vi "Init Hardware.vi"(8 "error in (no error)":errorcluster, 11 "Ni-Scope Digitizer in":refnum<class "Ni-Scope Digitizer.lvclass">) -> (0 "error out":errorcluster, 3 "Ni-Scope Digitizer out":refnum<class "Ni-Scope Digitizer.lvclass">)   [LabVIEW 2016, in "Ni-Scope Digitizer.lvclass"]
uses:
  Ni-Scope Digitizer.lvclass
  C:/github/NHMFL_Core/Libraries/Instruments/Pulse Driver/Pulse Driver.lvclass
  <instrlib>/niScope/Controls/niScope trigger source digital.ctl
  Ni-Scope Digitizer.lvclass/Ni-Scope Digitizer.ctl
  Instruments/Pulse Driver/Pulse Driver.lvclass/Pulse Driver.ctl
  Read Device name.vi
  Instruments/Pulse Driver/Read Pretrigger samples.vi
  Instruments/Pulse Driver/Read Samples per channel.vi
  Instruments/Pulse Driver/Write Samples per channel.vi
  Instruments/Pulse Driver/Write dt.vi
  Instruments/Pulse Driver/Write t0.vi
  <instrlib>/niScope/Configure/Trigger/niScope Configure Trigger Digital.vi
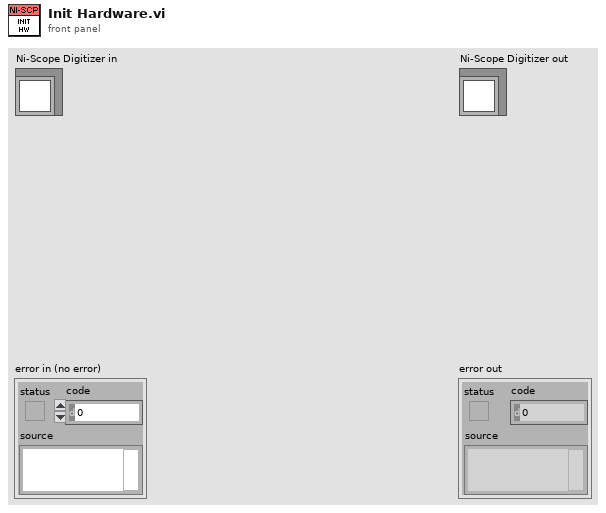
[diagram p1: front panel]
types:
  T1 = typedef "niScope trigger source digital.ctl" = string
  T2 = typedef "Pusle Driver Configuration.ctl" = cluster{"Pre-trigger duration":dbl, "Post-trigger duration":dbl, "Rate":dbl, "Ranges":dbl[], "Re-name channels":string[], "Active channels":string, "External clock":bool}
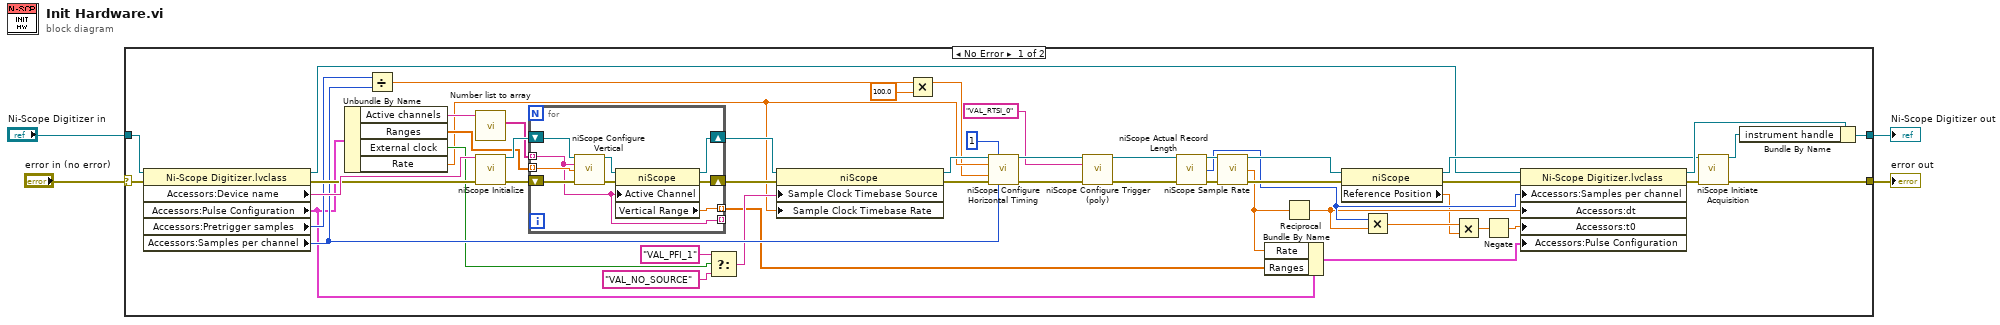
[diagram p0: block diagram]
diagram:
  n1 = case shown="No Error" "error in (no error)" {
    selector: "error in (no error)" -> [w44 w66]
    tunnel: [w8 w66] -> w3
    tunnel: [w14 w65] -> w1
    tunnel: "Ni-Scope Digitizer in" -> [w12 w65]
    frame No Error {
      n2 = property class="Ni-Scope Digitizer.lvclass"(reference=w12, error in=w44) -> (reference out=w11:refnum<class "Ni-Scope Digitizer.lvclass">, error out=w45:errorcluster, "Accessors:Device name"=w46:string, "Accessors:Pulse Configuration"=w26:T2, "Accessors:Pretrigger samples"=w42:u32, "Accessors:Samples per channel"=w43:i32)
      n3 = Unbundle By Name(w26) -> ("Active channels"=w49:string, "Ranges"=w47:dbl[], "External clock"=w37:bool, "Rate"=w33:dbl)
      n4 = Divide(x=w42, y=w43) -> (x/y=w52:dbl)
      n5 = call "Number list to array.vi"("Number list"=w49) -> ("Full names"=w48:string[])  [unwired: 9 in, 1 out]
      n6 = call <instrlib>:"niScope Initialize.vi"("resource name"=w46, "error in"=w45) -> ("instrument handle"=w54:refnum<k15>, "error out"=w55:errorcluster)  [unwired: 2 in, 10 out]
      n7 = for {
        tunnel: w47 -> [w62] mode=indexing
        shift-right: [w58] -> w40
        shift-left: w55 -> [w64]
        shift-right: [w60] -> w41
        shift-left: w54 -> [w63]
        tunnel: w48 -> [w57] mode=indexing
        tunnel: [w57] -> _ mode=indexing
        tunnel: [w56] -> w10 mode=indexing
        n8 = call <instrlib>:"niScope Configure Vertical.vi"("instrument handle"=w63, "channels"=w57, "vertical range"=w62, "error in"=w64) -> ("instrument handle out"=w61:refnum<k15>, "error out"=w59:errorcluster)  [unwired: 10 in]
        n9 = property class="niScope"(reference=w61, error in=w59, "Active Channel"=w57) -> (reference out=w60:refnum<k15>, error out=w58:errorcluster, "Vertical Range"=w56:dbl)
      }
      n10 = Select(t="VAL_PFI_1", s=w37, f="VAL_NO_SOURCE") -> (s? t:f=w34:string)
      n11 = property class="niScope"(reference=w41, error in=w40, "Sample Clock Timebase Source"=w34, "Sample Clock Timebase Rate"=w33) -> (reference out=w39:refnum<k15>, error out=w38:errorcluster)
      n12 = Multiply(x=w52, y=100.0) -> (x*y=w6:dbl)
      n13 = call <instrlib>:"niScope Configure Horizontal Timing.vi"("instrument handle"=w39, "number of records"=1, "min sample rate"=w33, "reference position"=w6, "error in"=w38, "min record length"=w43) -> ("instrument handle out"=w51:refnum<k15>, "error out"=w50:errorcluster)  [unwired: 1 in, 7 out]
      n14 = call-poly <instrlib>:"niScope Configure Trigger (poly).vi"("instrument handle"=w51, "trigger source"=T1 "VAL_RTSI_0", "error in"=w50) -> ("instrument handle out"=w30:refnum<k15>, "error out"=w31:errorcluster)  [unwired: 4 in, 7 out]
      n15 = call <instrlib>:"niScope Actual Record Length.vi"("instrument handle"=w30, "error in"=w31) -> ("instrument handle out"=w27:refnum<k15>, "actual record length"=w21:i32, "error out"=w28:errorcluster)  [unwired: 11 out]
      n16 = call <instrlib>:"niScope Sample Rate.vi"("instrument handle"=w27, "error in"=w28) -> ("instrument handle out"=w25:refnum<k15>, "actual sample rate"=w23:dbl, "error out"=w24:errorcluster)  [unwired: 11 out]
      n17 = Bundle By Name(cluster=w26, "Rate"=w23, "Ranges"=w10) -> (w22:T2)
      n18 = Reciprocal(x=w23) -> (1/x=w20:dbl)
      n19 = property class="niScope"(reference=w25, error in=w24) -> (reference out=w13:refnum<k15>, error out=w15:errorcluster, "Reference Position"=w18:dbl)
      n20 = Multiply(x=w21, y=w20) -> (x*y=w19:dbl)
      n21 = Multiply(x=w19, y=w18) -> (x*y=w17:dbl)
      n22 = Negate(x=w17) -> (-x=w16:dbl)
      n23 = property class="Ni-Scope Digitizer.lvclass"(reference=w11, error in=w15, "Accessors:Samples per channel"=w21, "Accessors:dt"=w20, "Accessors:t0"=w16, "Accessors:Pulse Configuration"=w22) -> (reference out=w29:refnum<class "Ni-Scope Digitizer.lvclass">, error out=w7:errorcluster)
      n24 = call <instrlib>:"niScope Initiate Acquisition.vi"("instrument handle"=w13, "error in"=w7) -> ("instrument handle out"=w9:refnum<k15>, "error out"=w8:errorcluster)  [unwired: 12 in]
      n25 = Bundle By Name(cluster=w29, "instrument handle"=w9) -> (w14:refnum<class "Ni-Scope Digitizer.lvclass">)
    }
    frame Error {
    }
  }
  "error out" <- w3
  "Ni-Scope Digitizer out" <- w1
